vi "ReadFpgaData.vi"(0 "Stand":refnum<class "Stand.lvclass">, 11 "error in (no error)":errorcluster) -> (4 "Stand out":refnum<class "Stand.lvclass">, 14 "dt":u32, 15 "error out":errorcluster)   [LabVIEW 2019, in "Stand.lvclass"]
uses:
  Stand.lvclass
  C:/Users/ANENKOV_V1/Desktop/src/Device_class/Device.lvclass
  FPGA/TypeDef/DO index.ctl
  Device_class/Device.lvclass/Device.ctl
  Stand.lvclass/Stand.ctl
  AI_class/AI.lvclass/AI.ctl
  PiecedLinearScale_class/Scale_PiecedLinear.lvclass/Scale_PiecedLinear.ctl
  Proccess_class/Proccess.lvclass/Proccess.ctl
  Logger_class/Logger.lvclass/Logger.ctl
  AnalogComparator_class/AnalogComparator.lvclass/AnalogComparator.ctl
  DI_class/DI.lvclass/DI.ctl
  DO_class/DO.lvclass/DO.ctl
  AO_class/AO.lvclass/AO.ctl
  FPGA_API_class/FPGA API.lvclass/FPGA API.ctl
  AI_class/SetRaw.vi
  DI_class/private/SendToDb.vi
  DO_class/private/SendToDb.vi
  AO_class/private/WriteToDb.vi
  Device_class/Write FPGA API.vi
  FPGA_API_class/Write Nitro.vi
  PiecedLinearScale_class/RawToScaled.vi
  subvis/Average.vi
  subvis/Loop Time Const.vi
  AI_class/HandleRanges.vi
  AI_class/HandleAlarms.vi
  AI_class/private/WriteToDb.vi
  Proccess_class/GetNames.vi
  Proccess_class/GetLogger.vi
  Logger_class/Enqueue Signal.vi
  AI_class/AI.lvclass
  C:/Users/ANENKOV_V1/Desktop/src/Proccess_class/Proccess.lvclass
  DI_class/DI.lvclass
  DO_class/DO.lvclass
  AO_class/AO.lvclass
  <vilib>/Analysis/baseanly.llb/Std Deviation and Variance.vi
  <vilib>/gmath/interp.llb/Interpolate 1D.vi
  <vilib>/Utility/error.llb/Error Cluster From Error Code.vi
  AnalogComparator_class/SendToDb.vi
  Logger_class/WriteEvent.vi
  FPGA_API_class/FPGA API.lvclass
  Device_class/Device.lvclass
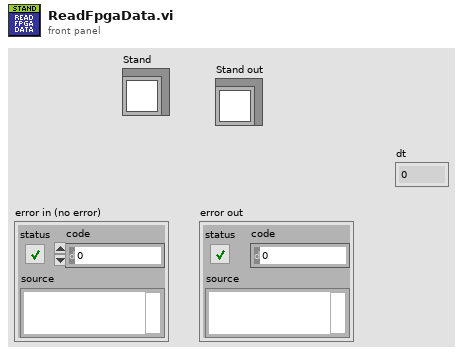
[diagram p1: front panel]
types:
  T1 = typedef "DO index.ctl" = u8
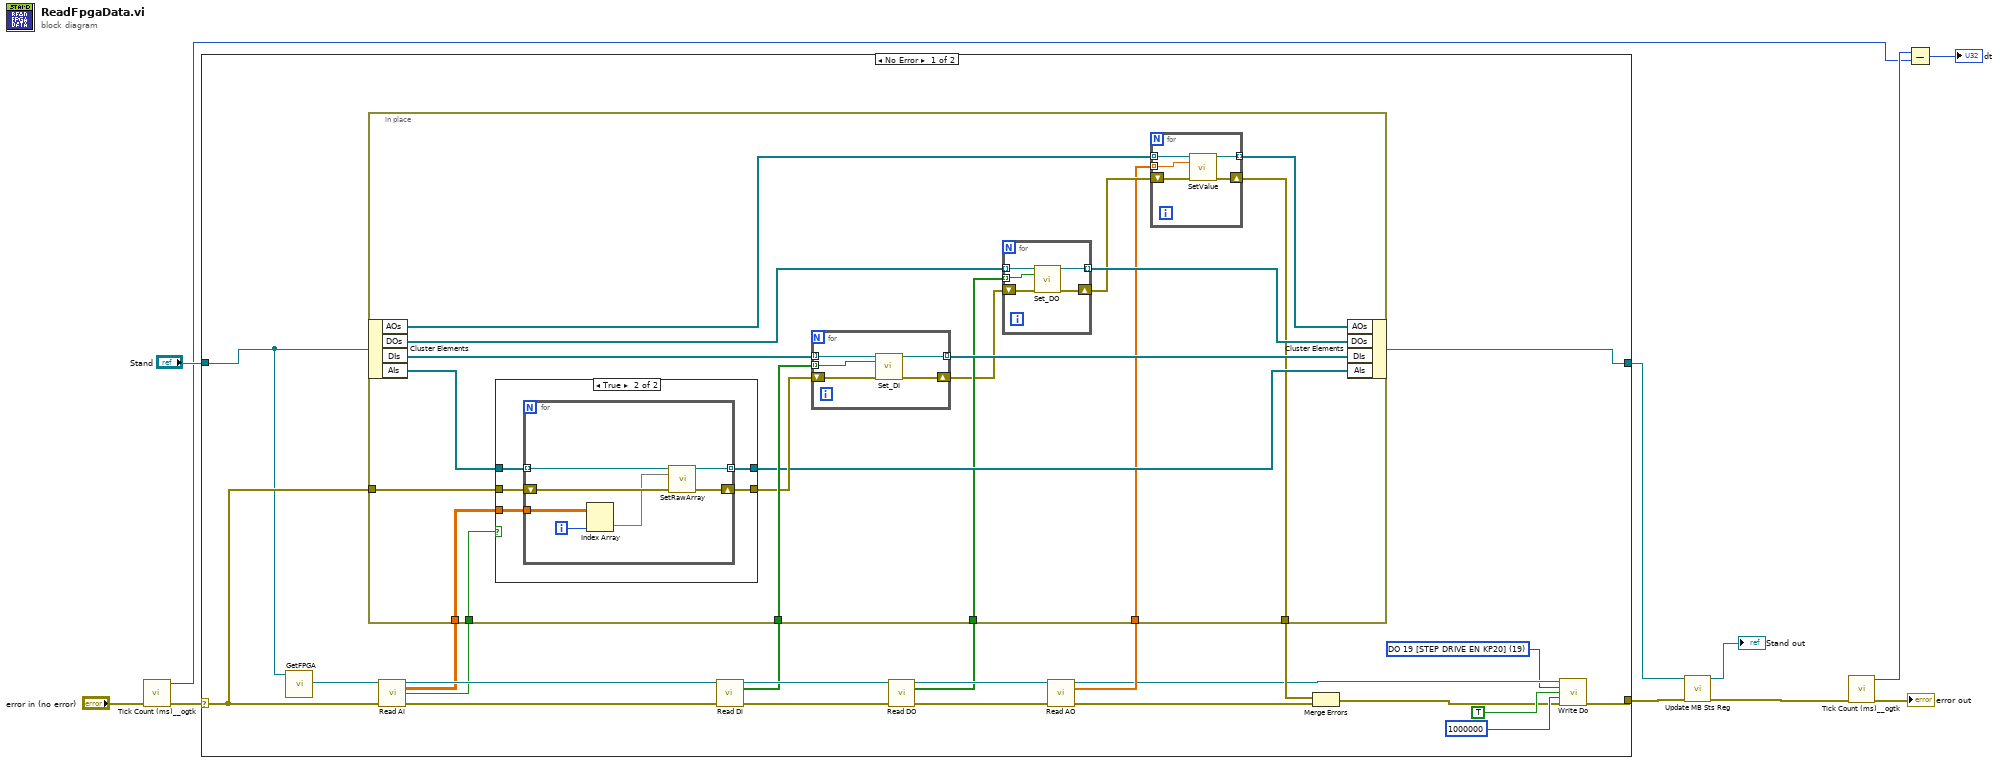
[diagram p0: block diagram]
diagram:
  n1 = call <userlib>:"Tick Count (ms)__ogtk.vi"("error in (no error)"="error in (no error)") -> ("error out"=w8:errorcluster, "millisecond timer value"=w4:u32)  [unwired: 9 in]
  n2 = case shown="No Error" w8 {
    selector: w8 -> [w32 w83]
    tunnel: "Stand" -> [w27 w82]
    tunnel: [w13 w83] -> w7
    tunnel: [w33 w82] -> w10
    frame No Error {
      w12 = T1 19 items=["DO 0 [KP1] [M12]", "DO 1 [ON KP2] [M21]", "DO 2 [ON KP3] [M24]", "DO 3 [WATER Y18.1 [DO3]]", "DO 4 [WATER Y18.2 [DO4]]", "DO 5 [KP6 Y29.1 33.7]", "DO 6 [KP7 Y29.2 33.8]", "DO 7 [KP8 Y29.3 33.9]", "DO 8 [KP9 Y29.4  33.12]", "DO 9 [KP10 Y29.5 33.1]", "DO 10 [KP11 Y29.6 33.2]", "DO 11 [KP12 Y29.7  33.13]", "DO 12 [KP13 Y29.8  33.11]", "DO 13 [KP14 Y29.9 33.10]", "DO 14 [KP15 Y29.10  33.6]", "DO 15 [KP16 Y29.11  33.5]", "DO 16 [KP17 Y29.12  33.4]", "DO 17 [KP18 Y29.13 33.3]", "DO 18 [AIR KP19]", "DO 19 [STEP DRIVE EN KP20]", "DO 20 [KP21 Y44.1 OPEN]", "DO 21 [ KP22 Y44.1 CLOSE]", "DO 22 [ KP23 Y44.2 OPEN]", "DO 23", "DO 24 [STEP DRIVE 1]", "DO 25 [STEP DRIVE 2]"] ("#DO")
      n3 = call "GetFPGA.vi"("Device in"=w27) -> ("FPGA API.lvclass"=w19:refnum<class "FPGA API.lvclass">)  [unwired: 10 in]
      n4 = call-dynamic "Read Ai.vi"("FPGA API in"=w19, "error in (no error)"=w32) -> ("FPGA API out"=w31:refnum<class "FPGA API.lvclass">, "AI Data"=w28:dbl[][], "Valud Data"=w29:bool, "error out"=w30:errorcluster)  [unwired: 10 in]
      n5 = call-dynamic "Read Di.vi"("FPGA API in"=w31, "error in (no error)"=w30) -> ("FPGA API out"=w25:refnum<class "FPGA API.lvclass">, "DIs"=w21:bool[], "error out"=w26:errorcluster)  [unwired: 11 in]
      n6 = call-dynamic "Read DO.vi"("FPGA API in"=w25, "error in (no error)"=w26) -> ("FPGA API out"=w20:refnum<class "FPGA API.lvclass">, "Ds"=w18:bool[], "error out"=w24:errorcluster)  [unwired: 11 in]
      n7 = call-dynamic "Read AO.vi"("FPGA API in"=w20, "error in (no error)"=w24) -> ("FPGA API out"=w15:refnum<class "FPGA API.lvclass">, "AO"=w22:dbl[], "error out"=w23:errorcluster)  [unwired: 11 in]
      n8 = in-place {
        in-place-border: w21 -> [w52]
        in-place-border: w32 -> [w49]
        in-place-border: [w36] -> w34
        in-place-border: w29 -> [w45]
        in-place-border: w28 -> [w44]
        in-place-border: w18 -> [w42]
        in-place-border: w22 -> [w35]
        n9 = in-place-cluster #1(w27) -> ("AOs"=w39:refnum<class "AO.lvclass">[], "DOs"=w43:refnum<class "DO.lvclass">[], "DIs"=w50:refnum<class "DI.lvclass">[], "AIs"=w51:refnum<class "AI.lvclass">[])
        n10 = case shown="True" w45 {
          tunnel: w51 -> [w69 w74]
          tunnel: w49 -> [w68 w73]
          tunnel: [w68 w72] -> w48
          tunnel: [w69 w71] -> w47
          tunnel: w44 -> [_ w70]
          frame False {
          }
          frame True {
            n11 = for {
              tunnel: w70 -> [w78]
              shift-right: [w80] -> w72
              shift-left: w73 -> [w79]
              tunnel: w74 -> [w77] mode=indexing
              tunnel: [w81] -> w71 mode=indexing
              i -> [w75]
              n12 = Index Array(array=w78, index (col)=w75) -> (element=w76:dbl[])  [unwired: 1 in]
              n13 = call "SetRawArray.vi"("reference in"=w77, "RAW"=w76, "error in (no error)"=w79) -> ("reference out"=w81:refnum<class "AI.lvclass">, "error out"=w80:errorcluster)  [unwired: 11 in]
            }
          }
        }
        n14 = for {
          tunnel: w50 -> [w67] mode=indexing
          tunnel: w52 -> [w66] mode=indexing
          shift-right: [w64] -> w41
          shift-left: w48 -> [w65]
          tunnel: [w63] -> w46 mode=indexing
          n15 = call "Set_DI.vi"("reference in"=w67, "DI"=w66, "error in (no error)"=w65) -> ("reference out"=w63:refnum<class "DI.lvclass">, "error out"=w64:errorcluster)  [unwired: 11 in]
        }
        n16 = for {
          tunnel: w43 -> [w62] mode=indexing
          tunnel: w42 -> [w61] mode=indexing
          shift-right: [w59] -> w37
          shift-left: w41 -> [w60]
          tunnel: [w58] -> w40 mode=indexing
          n17 = call "Set_DO.vi"("reference in"=w62, "DO"=w61, "error in (no error)"=w60) -> ("reference out"=w58:refnum<class "DO.lvclass">, "error out"=w59:errorcluster)  [unwired: 11 in]
        }
        n18 = for {
          tunnel: w39 -> [w57] mode=indexing
          tunnel: [w56] -> w38 mode=indexing
          shift-right: [w54] -> w36
          shift-left: w37 -> [w55]
          tunnel: w35 -> [w53] mode=indexing
          n19 = call "SetValue.vi"("reference in"=w57, "value"=w53, "error in (no error)"=w55) -> ("reference out"=w56:refnum<class "AO.lvclass">, "error out"=w54:errorcluster)  [unwired: 11 in]
        }
        n20 = in-place-cluster #1("AOs"=w38, "DOs"=w40, "DIs"=w46, "AIs"=w47) -> (w33:refnum<class "Stand.lvclass">)
      }
      n21 = Merge Errors(w34, w23) -> (w14:errorcluster)
      n22 = call-dynamic "Write Do.vi"("FPGA API in"=w15, "#DO"=w12, "value"=TRUE, "Time uSec"=u32 1000000, "error in (no error)"=w14) -> ("error out"=w13:errorcluster)  [unwired: 9 in, 1 out]
    }
    frame Error {
    }
  }
  n23 = call "Update MB Sts Reg.vi"("error in (no error)"=w7, "Stand in"=w10) -> ("error out"=w1:errorcluster, "Stand out"=→"Stand out":refnum<class "Stand.lvclass">)  [unwired: 8 in]
  n24 = call <userlib>:"Tick Count (ms)__ogtk.vi"("error in (no error)"=w1) -> ("error out"=→"error out":errorcluster, "millisecond timer value"=w5:u32)  [unwired: 9 in]
  n25 = Subtract(x=w5, y=w4) -> (x-y=→"dt":u32)
